vi "Calculate possible moves.vi"(7 "Position":refnum<class "Position.lvclass">, 8 "error in (no error)":errorcluster, 10 "Source":T1={"File"=enum."d", "Rank"=enum."4"}, 11 "Knight in":refnum<class "Knight.lvclass">) -> (0 "error out":errorcluster, 2 "Moves":refnum<class "Move.lvclass">[](array[class]), 3 "Knight out":refnum<class "Knight.lvclass">)   [LabVIEW 2016, in "Chesslib.lvlib" / "Knight.lvclass"]
uses:
  Knight.lvclass
  C:/Users/GRTaggJ/Documents/Projects/chesslib/Pieces/Piece/Piece.lvclass
  Moves/Move/Move.lvclass
  typedef/Square.ctl
  typedef/File.ctl
  typedef/Rank.ctl
  Position/Position.lvclass
  Position/Position.lvclass/Position.ctl
  Piece/Piece.lvclass/Piece.ctl
  Chesslib.lvlib
  Board/Board.lvclass
  Piece/Piece.lvclass
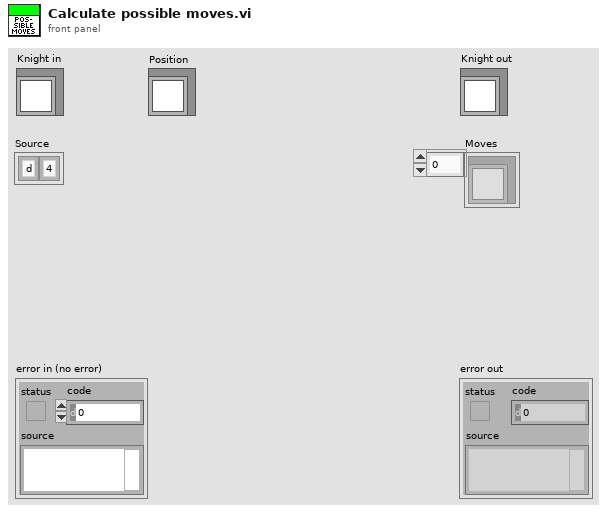
[diagram p1: front panel]
types:
  T1 = typedef "Chesslib.lvlib/Square.ctl" = cluster{"File":T2, "Rank":T3}
  T2 = typedef "Chesslib.lvlib/File.ctl" = enum8{"a", "b", "c", "d", "e", "f", "g", "h"}
  T3 = typedef "Chesslib.lvlib/Rank.ctl" = enum8{"1", "2", "3", "4", "5", "6", "7", "8"}
  T4 = typedef "Chesslib.lvlib/Color.ctl" = enum16{"White", "Black"}
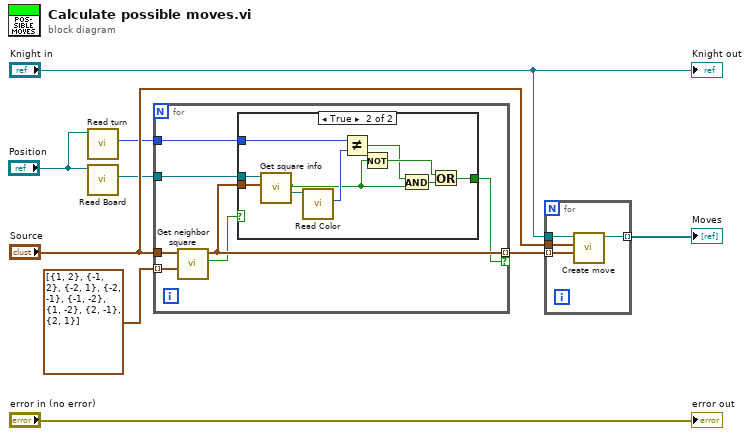
[diagram p0: block diagram]
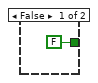
[diagram p2: hidden frame]
diagram:
  n1 = call "Read turn.vi"("Position in"="Position") -> ("Turn"=w2:T4)  [unwired: 9 in, 1 out]
  n2 = call "Read Board.vi"("Position in"="Position") -> ("Board"=w1:refnum<class "Board.lvclass">)  [unwired: 9 in, 1 out]
  n3 = for {
    tunnel: "Source" -> [w14]
    tunnel: cluster{i8, i8}[] [{1, 2}, {-1, 2}, {-2, 1}, {-2, -1}, {-1, -2}, {1, -2}, {2, -1}, {2, 1}] -> [w16] mode=indexing
    tunnel: [w13] -> w7 mode=indexing if=w10
    tunnel: w2 -> [w12]
    tunnel: w1 -> [w15]
    n4 = call "Get neighbor square.vi"("Vector (0, 0)"=w16, "Square in"=w14) -> ("Valid"=w11:bool, "Square out"=w13:T1)  [unwired: 8 in]
    n5 = case shown="True" w11 {
      tunnel: w15 -> [_ w27]
      tunnel: w13 -> [_ w25]
      tunnel: w12 -> [_ w23]
      tunnel: [FALSE w18] -> w10
      frame False {
      }
      frame True {
        n6 = call "Get square info.vi"("Square"=w25, "Board in"=w27) -> ("Piece"=w26:refnum<class "Piece.lvclass">, "Square occupied?"=w20:bool)  [unwired: 7 in, 1 out]
        n7 = call "Read Color.vi"("Piece in"=w26) -> ("Color"=w24:T4)  [unwired: 10 in]
        n8 = Not Equal?(x=w23, y=w24) -> (x != y?=w19:bool)
        n9 = Not(x=w20) -> (.not. x?=w22:bool)
        n10 = And(x=w19, y=w20) -> (x .and. y?=w21:bool)
        n11 = Or(x=w22, y=w21) -> (x .or. y?=w18:bool)
      }
    }
  }
  n12 = for {
    tunnel: w7 -> [w31] mode=indexing
    tunnel: "Source" -> [w30]
    tunnel: "Knight in" -> [w29]
    tunnel: [w28] -> w4 mode=indexing
    n13 = call "Create move.vi"("Destination"=w31, "Source"=w30, "Piece"=w29) -> ("Move out"=w28:refnum<class "Move.lvclass">)  [unwired: 8 in]
  }
  "Moves" <- w4
  "error out" <- "error in (no error)"
  "Knight out" <- "Knight in"
